vi "Constants.vi"() -> ()   [LabVIEW 2019, in "Globals.lvlib"]
doc: "Constant values either set statically in this global, or set once within Dataflow DJ."
uses:
  Globals.lvlib
panel:
  in  "Ramp (Fade Out)":dbl[](array[numeric])
  in  "Ramp (Fade In)":dbl[](array[numeric])
  in  "Waveform Graph Width":i32=523
  in  "Depth":i32=16
  in  "Channels":i32=2
  in  "Output Buffer Size":i32=1024
  in  "Zero Buffer":dbl[][](array[numeric])
  in  "Buffer Size":i32=1024
  in  "Sample Rate":i32=44100
  # "Sample Rate - Audio device output sample rate. All internal audio processing is done at this rate.\nChannels - Number of output channels\nDepth - Bit depth of audio output"
  # "Buffer Size - Size of internal audio processing buffer. Not necessarily the same as the output buffer, could be smaller for lower latency.\nOutput Buffer Size - Audio device output buffer size. Should be large enough to prevent audio drop-outs.\n\nIf using WaveIO, these buffers must be the same size."
  # "Zero Buffer - A block of memory init to Channels x Buffer Size. This is used when no real audio data is needed or available (no track loaded, track paused, etc)."
  # "Ramp (Fade In) - A block of memory init to Buffer Size, where the samples are a linear ramp from 0 to 1. This is used to apply an amplitude envelope to an audio block."
  # "Ramp (Fade Out) - A block of memory init to Buffer Size, where the samples are a linear ramp from 1 to 0. This is used to apply an amplitude envelope to an audio block."
  # "Waveform Graph Width - The width in pixels of the draw area of the waveform graph display. This number is used to calc the number of elements to display in the waveform."
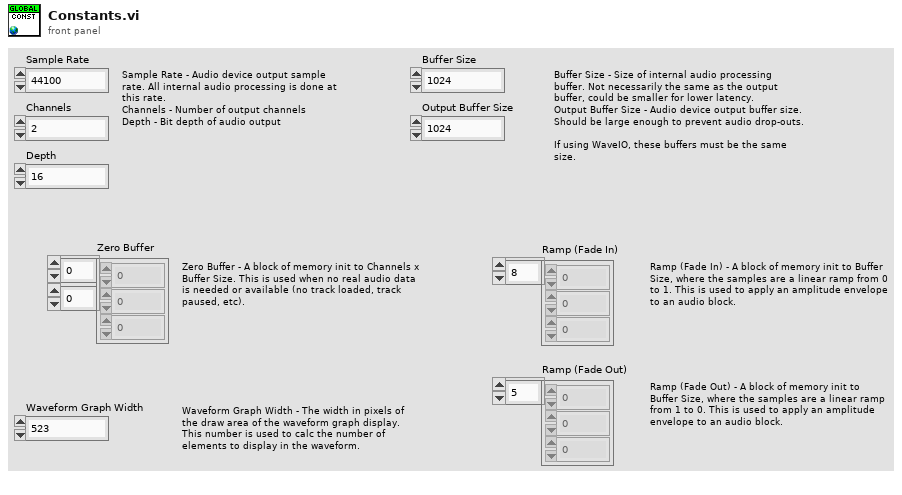
[diagram p1: front panel]
diagram:
